vi "GV RescanGalvoDelay_tick.vi"() -> ()   [LabVIEW 2017]
panel:
  out "RescanGalvoDelay_tick":u32
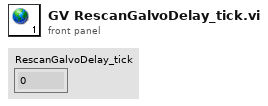
[diagram p1: front panel]
diagram:
